vi "pitot_dP.vi"(0 "Pitot Current":dynamicdata(graph), 1 "Pitot Offset [Pa]":dbl) -> (2 "dP H2O":dbl[](array[numeric]), 3 "dP [Pa]":dbl, 4 "Adj dP [Pa]":dbl, 5 "Adj dP [Pa] Array":dynamicdata(graph))   [LabVIEW 2017]
uses:
  <vilib>/express/express shared/transition.llb/Dynamic To Waveform Array.vi
  <vilib>/express/express arith-compare/Formula/Block/exnFormulaBlock how many pts in the wave.vi
  <vilib>/express/express shared/ex_Modify Signal Name.vi
  <vilib>/express/express shared/transition.llb/Waveform Array To Dynamic.vi
  <vilib>/express/express arith-compare/Formula/XNode/ExpressFormulaBlockNode.xnode
panel:
  in  "Pitot Current":i32
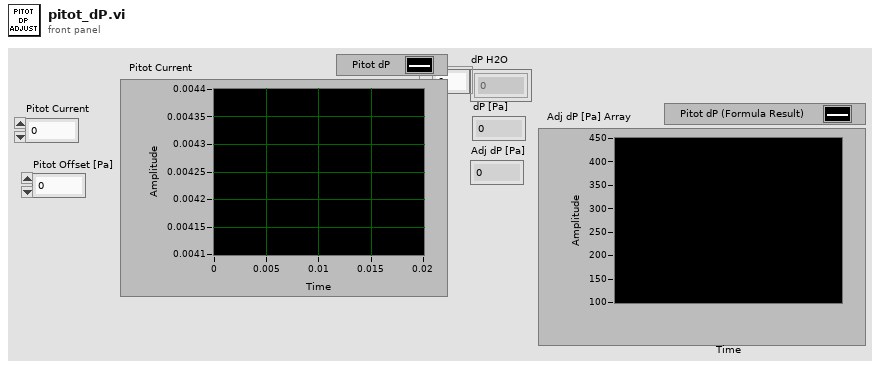
[diagram p1: front panel]
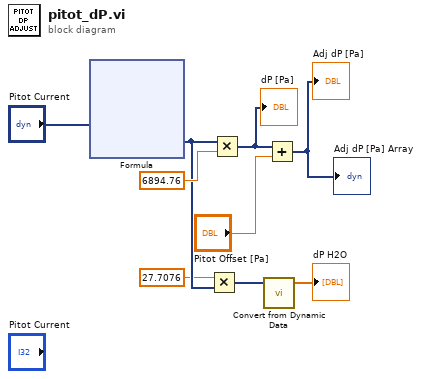
[diagram p0: block diagram]
diagram:
  n1 = xnode "Formula"("I"="Pitot Current") -> ("Result"=w5:dynamicdata)  [unwired: 1 in, 1 out]
  n2 = Multiply(x=27.7076, y=w5) -> (x*y=w6:dynamicdata)
  n3 = Multiply(x=w5, y=6894.76) -> (x*y=w8:dynamicdata)
  "dP [Pa]" <- w8
  n4 = call "Convert from Dynamic Data"("Dynamic Data Type"=w6) -> ("Array"=→"dP H2O":dbl[])  [unwired: 3 in]
  n5 = Add(x=w8, y="Pitot Offset [Pa]") -> (x+y=→"Adj dP [Pa]" →"Adj dP [Pa] Array":dynamicdata)
